vi "test_DMA Channels.vi"(8 "error in (no error)":errorcluster, 11 "TestCase in":refnum<class "DMA Channel Testing.lvclass">) -> (0 "error out":errorcluster, 3 "TestCase out":refnum<class "DMA Channel Testing.lvclass">)   [LabVIEW 2019, in "DMA Channel Testing.lvclass"]
uses:
  DMA Channel Testing.lvclass
  <vilib>/Utility/sysdir.llb/System Directory Type.ctl
  <vilib>/addons/_JKI Toolkits/VI Tester/TestCase.llb/TestCase.lvclass
  <vilib>/NI VeriStand/Execution/Workspace/NI_VS Workspace ExecutionAPI.lvlib
  C:/Program Files (x86)/National Instruments/LabVIEW 2019/vi.lib/addons/_JKI Toolkits/VI Tester/TestCase.llb/TestCase.lvclass
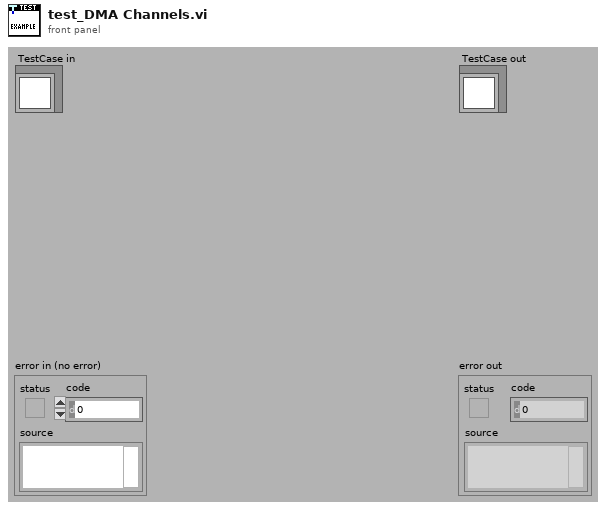
[diagram p1: front panel]
types:
  T1 = typedef "System Directory Type.ctl" = i32
  T2 = typedef "NI_VS Workspace ExecutionAPI.lvlib/WorkspaceAPI.ctl" = refnum<k24>
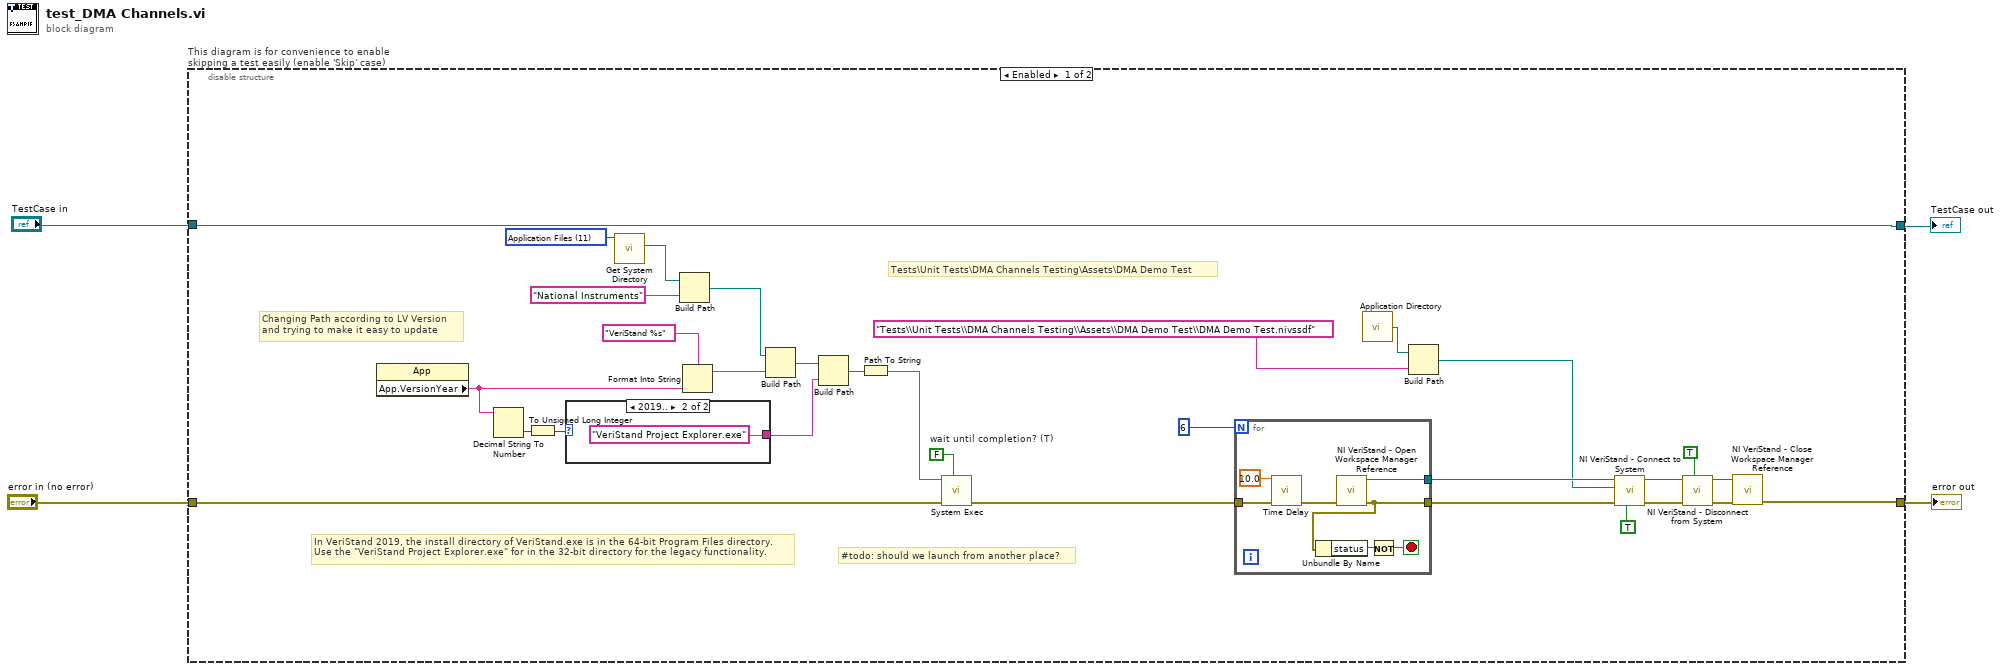
[diagram p0: block diagram]
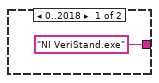
[diagram p2: hidden frame]
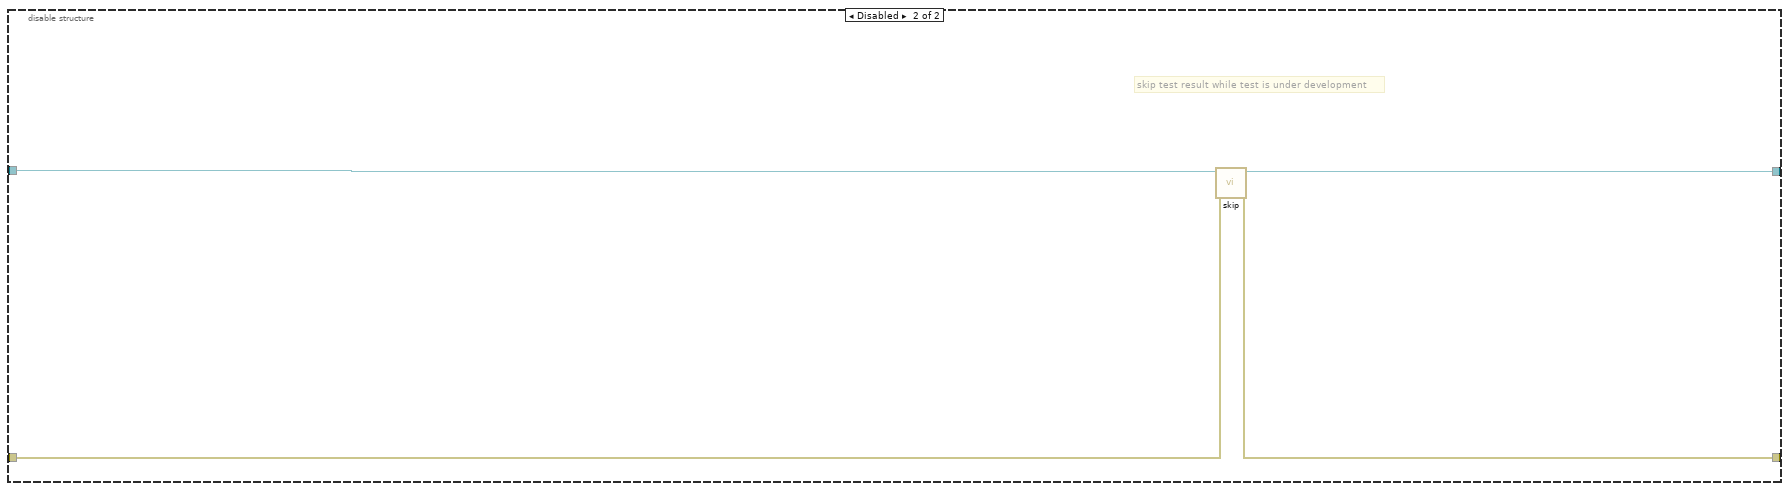
[diagram p3: hidden frame]
diagram:
  n1 = disable-structure "This diagram is for convenience to enable skipping a test easily (enable 'Skip' case)" shown="Enabled" {
    disable-tunnel: "TestCase in" -> [w28 w47]
    disable-tunnel: [w28 w45] -> w1
    disable-tunnel: [w29 w46] -> w3
    disable-tunnel: "error in (no error)" -> [w13 w44]
    frame Enabled {
      w22 = T1 11 items=["User Home"=0, "User Desktop"=1, "User Documents"=2, "User Application Data"=3, "User Preferences"=4, "User Temporary"=5, "Public Documents"=6, "Public Application Data"=7, "Public Preferences"=8, "Public Cache"=13, "System Core Libraries"=9, "System Installed Libraries"=10, "Application Files"=11, "Boot Volume Root"=12] ("system directory type")
      w27 = FALSE  # wait until completion? (T)
      # "Tests\\Unit Tests\\DMA Channels Testing\\Assets\\DMA Demo Test"
      # "In VeriStand 2019, the install directory of VeriStand.exe is in the 64-bit Program Files directory.\nUse the \"VeriStand Project Explorer.exe\" for in the 32-bit directory for the legacy functionality."
      # "Changing Path according to LV Version\nand trying to make it easy to update"
      # "#todo: should we launch from another place?"
      n2 = property class="App"() -> ("App.VersionYear"=w23:string)  [unwired: 2 in, 2 out]
      n3 = Decimal String To Number(string=w23) -> (number=w24:i32)  [unwired: 2 in, 1 out]
      n4 = To Unsigned Long Integer(number=w24) -> (unsigned 32bit integer=w14:u32)
      n5 = case shown="2019.." w14 {
        tunnel: ["NI VeriStand.exe" ("command line") "VeriStand Project Explorer.exe" ("command line")] -> w17
        frame 0..2018 {
        }
        frame 2019.. {
        }
      }
      n6 = call <vilib>:"Get System Directory.vi"("system directory type"=w22) -> ("system directory"=w20:path)  [unwired: 10 in]
      n7 = Build Path(base path=w20, name or relative path="National Instruments" ("command line")) -> (appended path=w19:path)
      n8 = Format Into String(format string="VeriStand %s" ("command line"), w23) -> (resulting string=w18:string)  [unwired: 2 in, 1 out]
      n9 = Build Path(base path=w19, name or relative path=w18) -> (appended path=w16:path)
      n10 = Build Path(base path=w16, name or relative path=w17) -> (appended path=w25:path)
      n11 = Path To String(path=w25) -> (string=w26:string)
      n12 = call <vilib>:"System Exec.vi"("wait until completion? (T)"=w27, "error in (no error)"=w13, "command line"=w26) -> ("error out"=w11:errorcluster)  [unwired: 5 in, 3 out]
      n13 = for {
        N: 6 -> [_]
        tunnel: [w41] -> w10
        tunnel: w11 -> [w39]
        tunnel: [w37] -> w9
        stop <- w35 stop-if-true
        n14 = call "Time Delay"("error in (no error)"=w39, "Delay Time (s)"=10.0) -> ("error out"=w38:errorcluster)  [unwired: 9 in]
        n15 = call <vilib>:"NI VeriStand - Open Workspace Manager Reference.vi"("error in (no error)"=w38) -> ("error out"=w37:errorcluster, "WorkspaceManager"=w41:T2)  [unwired: 9 in]
        n16 = Unbundle By Name(w37) -> ("status"=w36:bool)
        n17 = Not(x=w36) -> (.not. x?=w35:bool)
      }
      n18 = call <vilib>:"Application Directory.vi"() -> ("Application Directory"=w7:path)
      n19 = Build Path(base path=w7, name or relative path="Tests\\Unit Tests\\DMA Channels Testing\\Assets\\DMA Demo Test\\DMA Demo Test.nivssdf") -> (appended path=w6:path)
      n20 = call <vilib>:"NI VeriStand - Connect to System.vi"("Deploy System Definition (T)"=TRUE, "error in (no error)"=w9, "System Definition File (.nivssdf)"=w6, "WorkspaceManager in"=w10) -> ("error out"=w32:errorcluster, "WorkspaceManager out"=w31:T2)  [unwired: 6 in]
      n21 = call <vilib>:"NI VeriStand - Disconnect from System.vi"("Undeploy System Definition (F)"=TRUE, "error in (no error)"=w32, "WorkspaceManager in"=w31) -> ("error out"=w30:errorcluster, "WorkspaceManager out"=w33:T2)  [unwired: 7 in]
      n22 = call <vilib>:"NI VeriStand - Close Workspace Manager Reference.vi"("error in (no error)"=w30, "WorkspaceManager"=w33) -> ("error out"=w29:errorcluster)  [unwired: 9 in]
    }
    frame Disabled {
      # "skip test result while test is under development"
      n23 = call <vilib>:"skip.vi"("error in (no error)"=w44, "TestCase in"=w47) -> ("error out"=w46:errorcluster, "TestCase out"=w45:refnum<class "DMA Channel Testing.lvclass">)  [unwired: 8 in]
    }
  }
  "error out" <- w3
  "TestCase out" <- w1
